vi "LifetimeCalculation.vi"(9 "LaserRepRate":dbl=80000000.0, 10 "S":dbl[][](array[numeric]), 11 "G":dbl[][](array[numeric])) -> (2 "DC&1w Lifetime":dbl[][](array[numeric]), 3 "1w Lifetime":dbl[][](array[numeric]))   [LabVIEW 2018]
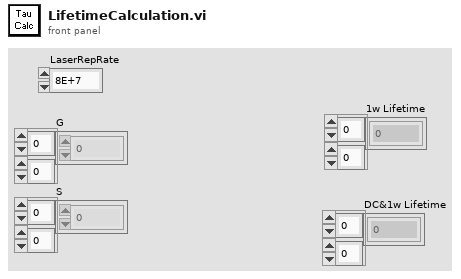
[diagram p1: front panel]
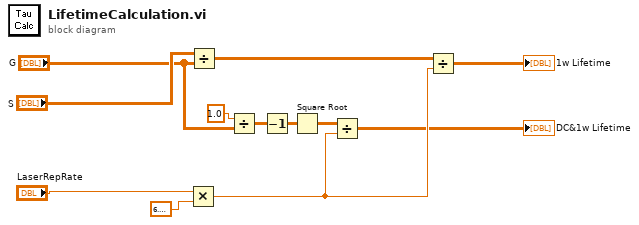
[diagram p0: block diagram]
diagram:
  n1 = Multiply(x="LaserRepRate", y=6.283185307179586) -> (x*y=w3:dbl)
  n2 = Divide(x="S", y="G") -> (x/y=w11:dbl[][])
  n3 = Divide(x=1.0, y="G") -> (x/y=w6:dbl[][])
  n4 = Decrement(x=w6) -> (x-1=w8:dbl[][])
  n5 = Square Root(x=w8) -> (sqrt(x)=w5:dbl[][])
  n6 = Divide(x=w5, y=w3) -> (x/y=→"DC&1w Lifetime":dbl[][])
  n7 = Divide(x=w11, y=w3) -> (x/y=→"1w Lifetime":dbl[][])
